vi "Lab Panel V5.22.vi"() -> ()   [LabVIEW 2013] (continued)
                            n2491 = Bundle By Name("Y"=w4658, "t0"=w4656) -> (w4650:waveform(dbl))  [unwired: 1 in]
                            n2492 = Bundle By Name("Y"=w4657, "t0"=w4656) -> (w4649:waveform(dbl))  [unwired: 1 in]
                            n2493 = Build Array(w4655, w4654, w4653, w4652, w4651, w4650, w4649) -> (w4648:waveform(dbl)[])
                            n2494 = TDMS Write(0:w4669, 5:"TEST VALUES", 7:w4640, 9:w4648) -> (4:w4639:refnum<k34>, 6:w4638:string, 15:w4637:errorcluster)  [unwired: 2 in, 1 out]
                            n2495 = TDMS Write(0:w4639, 5:w4638, 7:"TIME", 9:w4635, 11:w4637) -> (15:w4634:errorcluster)  [unwired: 1 in, 3 out]
                            n2496 = local write "data file error"(w4634) -> ()
                          }
                        }
                      }
                    }
                  }
                }
              }
            }
          }
          frame #13 {
            # "display test values on chart"
            n2497 = local read "jig cycle"() -> (w4677:dbl)
            n2498 = local read "on loops"() -> (w4679:dbl)
            n2499 = Add(x=w4679, y=2) -> (x+y=w4676:dbl)
            n2500 = Equal?(x=w4677, y=1) -> (x = y?=w4675:bool)
            n2501 = Equal?(x=w4677, y=w4676) -> (x = y?=w4674:bool)
            n2502 = Or(x=w4675, y=w4674) -> (x .or. y?=w4673:bool)
            "graph flag" <- w4673
            n2503 = global write "Global display 3.vi" "graph flag"(w4673) -> ()
            n2504 = case shown="True" w4673 {
              frame False {
              }
              frame True {
                n2505 = local read "SIG LAB05-1"() -> (w4722:T2)
                n2506 = local read "SIG LAB04-2"() -> (w4723:T2)
                n2507 = local read "SIG LAB05-2"() -> (w4721:T2)
                n2508 = local read "SIG LAB04-1"() -> (w4724:T2)
                n2509 = local read "SIG LAB03-1"() -> (w4726:T2)
                n2510 = local read "SIG LAB03-2"() -> (w4725:T2)
                n2511 = local read "SIG LAB01-1"() -> (w4730:T2)
                n2512 = local read "SIG LAB02-2"() -> (w4727:T2)
                n2513 = local read "SIG LAB02-1"() -> (w4728:T2)
                n2514 = local read "SIG LAB01-2"() -> (w4729:T2)
                n2515 = Unbundle(w4723) -> ("AMPS"=w4713:dbl, "VOLTS"=w4703:dbl, "Tmp Live"=w4693:dbl, "Tmp Neut"=w4683:dbl)  [unwired: 1 out]
                n2516 = Unbundle(w4722) -> ("AMPS"=w4712:dbl, "VOLTS"=w4702:dbl, "Tmp Live"=w4692:dbl, "Tmp Neut"=w4682:dbl)  [unwired: 1 out]
                n2517 = Unbundle(w4721) -> ("AMPS"=w4711:dbl, "VOLTS"=w4701:dbl, "Tmp Live"=w4691:dbl, "Tmp Neut"=w4681:dbl)  [unwired: 1 out]
                n2518 = Unbundle(w4724) -> ("AMPS"=w4714:dbl, "VOLTS"=w4704:dbl, "Tmp Live"=w4694:dbl, "Tmp Neut"=w4684:dbl)  [unwired: 1 out]
                n2519 = Unbundle(w4725) -> ("AMPS"=w4715:dbl, "VOLTS"=w4705:dbl, "Tmp Live"=w4695:dbl, "Tmp Neut"=w4685:dbl)  [unwired: 1 out]
                n2520 = Unbundle(w4726) -> ("AMPS"=w4716:dbl, "VOLTS"=w4706:dbl, "Tmp Live"=w4696:dbl, "Tmp Neut"=w4686:dbl)  [unwired: 1 out]
                n2521 = Unbundle(w4727) -> ("AMPS"=w4717:dbl, "VOLTS"=w4707:dbl, "Tmp Live"=w4697:dbl, "Tmp Neut"=w4687:dbl)  [unwired: 1 out]
                n2522 = Unbundle(w4728) -> ("AMPS"=w4718:dbl, "VOLTS"=w4708:dbl, "Tmp Live"=w4698:dbl, "Tmp Neut"=w4688:dbl)  [unwired: 1 out]
                n2523 = Unbundle(w4730) -> ("AMPS"=w4720:dbl, "VOLTS"=w4710:dbl, "Tmp Live"=w4700:dbl, "Tmp Neut"=w4690:dbl)  [unwired: 1 out]
                n2524 = Unbundle(w4729) -> ("AMPS"=w4719:dbl, "VOLTS"=w4709:dbl, "Tmp Live"=w4699:dbl, "Tmp Neut"=w4689:dbl)  [unwired: 1 out]
                n2525 = stacked-sequence {
                  tunnel: w4720 -> [w4762 _ _]
                  tunnel: w4719 -> [w4761 _ _]
                  tunnel: w4718 -> [w4752 _ _]
                  tunnel: w4717 -> [w4751 _ _]
                  tunnel: w4716 -> [w4741 _ _]
                  tunnel: w4715 -> [w4740 _ _]
                  tunnel: w4714 -> [_ w4785 _]
                  tunnel: w4713 -> [_ w4784 _]
                  tunnel: w4712 -> [_ w4774 _]
                  tunnel: w4711 -> [_ w4773 _]
                  tunnel: w4710 -> [w4759 _ _]
                  tunnel: w4709 -> [w4758 _ _]
                  tunnel: w4708 -> [w4749 _ _]
                  tunnel: w4707 -> [w4748 _ _]
                  tunnel: w4706 -> [w4739 _ _]
                  tunnel: w4705 -> [w4738 _ _]
                  tunnel: w4704 -> [_ w4783 _]
                  tunnel: w4703 -> [_ w4782 _]
                  tunnel: w4702 -> [_ w4772 _]
                  tunnel: w4701 -> [_ w4771 _]
                  tunnel: w4700 -> [w4756 _ _]
                  tunnel: w4699 -> [w4754 _ _]
                  tunnel: w4698 -> [w4745 _ _]
                  tunnel: w4697 -> [w4743 _ _]
                  tunnel: w4696 -> [w4737 _ _]
                  tunnel: w4695 -> [w4735 _ _]
                  tunnel: w4694 -> [_ w4781 _]
                  tunnel: w4693 -> [_ w4779 _]
                  tunnel: w4692 -> [_ w4770 _]
                  tunnel: w4691 -> [_ w4768 _]
                  tunnel: w4690 -> [w4755 _ _]
                  tunnel: w4689 -> [w4753 _ _]
                  tunnel: w4688 -> [w4744 _ _]
                  tunnel: w4687 -> [w4742 _ _]
                  tunnel: w4686 -> [w4736 _ _]
                  tunnel: w4685 -> [w4734 _ _]
                  tunnel: w4684 -> [_ w4780 _]
                  tunnel: w4683 -> [_ w4778 _]
                  tunnel: w4682 -> [_ w4769 _]
                  tunnel: w4681 -> [_ w4767 _]
                  frame #0 {
                    n2526 = Merge Signals(w4762, w4761) -> (→"LAB01 AMPS":dynamicdata)
                    n2527 = Merge Signals(w4759, w4758) -> (→"LAB01 VOLTS":dynamicdata)
                    n2528 = Merge Signals(w4739, w4738) -> (→"LAB03 VOLTS":dynamicdata)
                    n2529 = Merge Signals(w4756, w4755, w4754, w4753) -> (→"LAB01 deg C":dynamicdata)
                    n2530 = Merge Signals(w4752, w4751) -> (→"LAB02 AMPS":dynamicdata)
                    n2531 = Merge Signals(w4745, w4744, w4743, w4742) -> (→"LAB02 deg C":dynamicdata)
                    n2532 = Merge Signals(w4737, w4736, w4735, w4734) -> (→"LAB03 deg C":dynamicdata)
                    n2533 = Merge Signals(w4749, w4748) -> (→"LAB02 VOLTS":dynamicdata)
                    n2534 = Merge Signals(w4741, w4740) -> (→"LAB03 AMPS":dynamicdata)
                  }
                  frame #1 {
                    n2535 = Merge Signals(w4772, w4771) -> (→"LAB05 VOLTS":dynamicdata)
                    n2536 = Merge Signals(w4785, w4784) -> (→"LAB04 AMPS":dynamicdata)
                    n2537 = Merge Signals(w4774, w4773) -> (→"LAB05 AMPS":dynamicdata)
                    n2538 = Merge Signals(w4770, w4769, w4768, w4767) -> (→"LAB05 deg C":dynamicdata)
                    n2539 = Merge Signals(w4781, w4780, w4779, w4778) -> (→"LAB04 deg C":dynamicdata)
                    n2540 = Merge Signals(w4783, w4782) -> (→"LAB04 VOLTS":dynamicdata)
                  }
                  frame #2 {
                    n2541 = local read "LAB05 VOLTS"() -> (w4793:dynamicdata)
                    n2542 = local read "LAB04 VOLTS"() -> (w4794:dynamicdata)
                    n2543 = local read "LAB02 VOLTS"() -> (w4796:dynamicdata)
                    n2544 = local read "LAB03 VOLTS"() -> (w4795:dynamicdata)
                    n2545 = local read "LAB05 AMPS"() -> (w4799:dynamicdata)
                    n2546 = local read "LAB01 VOLTS"() -> (w4797:dynamicdata)
                    n2547 = local read "LAB04 AMPS"() -> (w4800:dynamicdata)
                    n2548 = local read "LAB03 AMPS"() -> (w4801:dynamicdata)
                    n2549 = local read "LAB03 deg C"() -> (w4789:dynamicdata)
                    n2550 = local read "LAB02 AMPS"() -> (w4802:dynamicdata)
                    n2551 = local read "LAB04 deg C"() -> (w4788:dynamicdata)
                    n2552 = local read "LAB05 deg C"() -> (w4787:dynamicdata)
                    n2553 = local read "LAB02 deg C"() -> (w4790:dynamicdata)
                    n2554 = local read "LAB01 deg C"() -> (w4791:dynamicdata)
                    n2555 = local read "LAB01 AMPS"() -> (w4803:dynamicdata)
                    n2556 = Merge Signals(w4791, w4790, w4789, w4788, w4787) -> (w4786:dynamicdata)
                    n2557 = Merge Signals(w4803, w4802, w4801, w4800, w4799) -> (w4798:dynamicdata)
                    n2558 = Merge Signals(w4797, w4796, w4795, w4794, w4793) -> (w4792:dynamicdata)
                    n2559 = global write "Global display 3.vi" "graph volts"(w4792) -> ()
                    n2560 = global write "Global display 3.vi" "graph deg C"(w4786) -> ()
                    n2561 = global write "Global display 3.vi" "graph amps"(w4798) -> ()
                  }
                }
              }
            }
          }
          frame #14 {
            # "check for amps fail"
            # "check for cycle test & temperature rise fail conditions"
            n2562 = local read "on loops"() -> (w4830:dbl)
            n2563 = local read "jig cycle"() -> (w4827:dbl)
            n2564 = local read "jig cycle"() -> (w4832:dbl)
            n2565 = Add(x=w4830, y=3.0) -> (x+y=w4828:dbl)
            n2566 = Equal?(x=w4827, y=w4828) -> (x = y?=w4823:bool)
            n2567 = local read "Fail Loops"() -> (w4804:dbl)
            n2568 = Equal?(x=w4832, y=1.0) -> (x = y?=w4825:bool)
            n2569 = global write "Global 1.vi" "fail count"(w4804) -> ()
            n2570 = stacked-sequence {
              tunnel: w4826 -> [w4835 _ _ _ _ _ _ _ _ _]
              tunnel: w4825 -> [w4836 w4856 w4876 w4896 w4916 w4936 w4956 w4976 w4996 w5016]
              tunnel: w4824 -> [w4833 _ _ _ _ _ _ _ _ _]
              tunnel: w4823 -> [w4834 w4855 w4875 w4895 w4915 w4935 w4955 w4975 w4995 w5015]
              tunnel: w4822 -> [_ w4854 _ _ _ _ _ _ _ _]
              tunnel: w4821 -> [_ w4853 _ _ _ _ _ _ _ _]
              tunnel: w4820 -> [_ _ w4874 _ _ _ _ _ _ _]
              tunnel: w4819 -> [_ _ w4873 _ _ _ _ _ _ _]
              tunnel: w4818 -> [_ _ _ w4894 _ _ _ _ _ _]
              tunnel: w4817 -> [_ _ _ w4893 _ _ _ _ _ _]
              tunnel: w4816 -> [_ _ _ _ w4914 _ _ _ _ _]
              tunnel: w4815 -> [_ _ _ _ w4913 _ _ _ _ _]
              tunnel: w4814 -> [_ _ _ _ _ w4934 _ _ _ _]
              tunnel: w4813 -> [_ _ _ _ _ w4933 _ _ _ _]
              tunnel: w4812 -> [_ _ _ _ _ _ w4954 _ _ _]
              tunnel: w4811 -> [_ _ _ _ _ _ w4953 _ _ _]
              tunnel: w4810 -> [_ _ _ _ _ _ _ w4974 _ _]
              tunnel: w4809 -> [_ _ _ _ _ _ _ w4973 _ _]
              tunnel: w4808 -> [_ _ _ _ _ _ _ _ w4994 _]
              tunnel: w4807 -> [_ _ _ _ _ _ _ _ w4993 _]
              tunnel: w4806 -> [_ _ _ _ _ _ _ _ _ w5014]
              tunnel: w4805 -> [_ _ _ _ _ _ _ _ _ w5013]
              frame #0 {
                # "LAB01-1"
                n2571 = case shown="True" w4833 {
                  tunnel: w4836 -> [_ w4849]
                  tunnel: w4835 -> [_ w4846]
                  tunnel: w4834 -> [_ w4845]
                  frame False {
                  }
                  frame True {
                    n2572 = local read "TEMP START LAB01-1"() -> (w4851:cluster{"TL":dbl, "TN":dbl})
                    n2573 = local read "RESULT LAB01-1"() -> (w4840:bool)
                    n2574 = local read "FAIL LAB01-1"() -> (w4843:cluster{"LO":dbl, "HI":dbl})
                    n2575 = local read "TDMS LAB01-1"() -> (w4850:refnum<k34>)
                    n2576 = local read "SET LAB01-1"() -> (w4847:T5)
                    n2577 = local read "DISP LAB01-1"() -> (w4848:T4)
                    n2578 = local read "SIG LAB01-1"() -> (w4852:T2)
                    n2579 = Bundle("FAIL LAB01-1"=w4843, "SIG LAB01-1"=w4852, "TEMP START LAB01-1"=w4851, "DISP LAB01-1"=w4848, "SET LAB01-1"=w4847, "TDMS LAB01-1"=w4850) -> (w4837:T32)  [unwired: 1 in]
                    n2580 = call "sub vi - cycle&temp fail v7.vi"("Amps Lo?"=w4849, "Input Cluster"=w4837, "SELECT"=w4846, "Amps Hi?"=w4845, "Result In"=w4840) -> ("(FAIL) out"=w4842:cluster{"FAIL LO":dbl, "FAIL HI":dbl}, "(DISP) out"=w4838:T4, "T-RISE"=w4839:cluster{"T-RISE (L)":dbl, "T-RISE (N)":dbl}, "Result Out"=w4841:bool, "file error"=w4844:errorcluster)  [unwired: 10 in]
                    n2581 = local write "TEMP RISE LAB01-1"(w4839) -> ()
                    n2582 = local write "FAIL LAB01-1"(w4842) -> ()
                    n2583 = local write "DISP LAB01-1"(w4838) -> ()
                    n2584 = local write "RESULT LAB01-1"(w4841) -> ()
                    n2585 = local write "data file error"(w4844) -> ()
                  }
                }
              }
              frame #1 {
                # "LAB01-2"
                n2586 = case shown="True" w4854 {
                  tunnel: w4856 -> [_ w4869]
                  tunnel: w4853 -> [_ w4866]
                  tunnel: w4855 -> [_ w4865]
                  frame False {
                  }
                  frame True {
                    n2587 = local read "TEMP START LAB01-2"() -> (w4871:cluster{"TL":dbl, "TN":dbl})
                    n2588 = local read "FAIL LAB01-2"() -> (w4862:cluster{"LO":dbl, "HI":dbl})
                    n2589 = local read "TDMS LAB01-2"() -> (w4870:refnum<k34>)
                    n2590 = local read "SET LAB01-2"() -> (w4867:T5)
                    n2591 = local read "DISP LAB01-2"() -> (w4868:T4)
                    n2592 = local read "RESULT LAB01-2"() -> (w4859:bool)
                    n2593 = local read "SIG LAB01-2"() -> (w4872:T2)
                    n2594 = Bundle("FAIL LAB01-2"=w4862, "SIG LAB01-2"=w4872, "TEMP START LAB01-2"=w4871, "DISP LAB01-2"=w4868, "SET LAB01-2"=w4867, "TDMS LAB01-2"=w4870) -> (w4857:T33)  [unwired: 1 in]
                    n2595 = call "sub vi - cycle&temp fail v7.vi"("Amps Lo?"=w4869, "Input Cluster"=w4857, "SELECT"=w4866, "Amps Hi?"=w4865, "Result In"=w4859) -> ("(FAIL) out"=w4861:cluster{"FAIL LO":dbl, "FAIL HI":dbl}, "(DISP) out"=w4864:T4, "T-RISE"=w4858:cluster{"T-RISE (L)":dbl, "T-RISE (N)":dbl}, "Result Out"=w4860:bool, "file error"=w4863:errorcluster)  [unwired: 10 in]
                    n2596 = local write "TEMP RISE LAB01-2"(w4858) -> ()
                    n2597 = local write "FAIL LAB01-2"(w4861) -> ()
                    n2598 = local write "DISP LAB01-2"(w4864) -> ()
                    n2599 = local write "RESULT LAB01-2"(w4860) -> ()
                    n2600 = local write "data file error"(w4863) -> ()
                  }
                }
              }
              frame #2 {
                # "LAB02-1"
                n2601 = case shown="True" w4874 {
                  tunnel: w4876 -> [_ w4889]
                  tunnel: w4873 -> [_ w4886]
                  tunnel: w4875 -> [_ w4885]
                  frame False {
                  }
                  frame True {
                    n2602 = local read "TEMP START LAB02-1"() -> (w4891:cluster{"TL":dbl, "TN":dbl})
                    n2603 = local read "FAIL LAB02-1"() -> (w4882:cluster{"LO":dbl, "HI":dbl})
                    n2604 = local read "TDMS LAB02-1"() -> (w4890:refnum<k34>)
                    n2605 = local read "SET LAB02-1"() -> (w4887:T5)
                    n2606 = local read "DISP LAB02-1"() -> (w4888:T4)
                    n2607 = local read "SIG LAB02-1"() -> (w4892:T2)
                    n2608 = local read "RESULT LAB02-1"() -> (w4879:bool)
                    n2609 = Bundle("FAIL LAB02-1"=w4882, "SIG LAB02-1"=w4892, "TEMP START LAB02-1"=w4891, "DISP LAB02-1"=w4888, "SET LAB02-1"=w4887, "TDMS LAB02-1"=w4890) -> (w4877:T34)  [unwired: 1 in]
                    n2610 = call "sub vi - cycle&temp fail v7.vi"("Amps Lo?"=w4889, "Input Cluster"=w4877, "SELECT"=w4886, "Amps Hi?"=w4885, "Result In"=w4879) -> ("(FAIL) out"=w4881:cluster{"FAIL LO":dbl, "FAIL HI":dbl}, "(DISP) out"=w4884:T4, "T-RISE"=w4878:cluster{"T-RISE (L)":dbl, "T-RISE (N)":dbl}, "Result Out"=w4880:bool, "file error"=w4883:errorcluster)  [unwired: 10 in]
                    n2611 = local write "TEMP RISE LAB02-1"(w4878) -> ()
                    n2612 = local write "FAIL LAB02-1"(w4881) -> ()
                    n2613 = local write "DISP LAB02-1"(w4884) -> ()
                    n2614 = local write "RESULT LAB02-1"(w4880) -> ()
                    n2615 = local write "data file error"(w4883) -> ()
                  }
                }
              }
              frame #3 {
                # "LAB02-2"
                n2616 = case shown="True" w4894 {
                  tunnel: w4896 -> [_ w4909]
                  tunnel: w4893 -> [_ w4906]
                  tunnel: w4895 -> [_ w4905]
                  frame False {
                  }
                  frame True {
                    n2617 = local read "TEMP START LAB02-2"() -> (w4911:cluster{"TL":dbl, "TN":dbl})
                    n2618 = local read "FAIL LAB02-2"() -> (w4902:cluster{"LO":dbl, "HI":dbl})
                    n2619 = local read "TDMS LAB02-2"() -> (w4910:refnum<k34>)
                    n2620 = local read "SET LAB02-2"() -> (w4907:T5)
                    n2621 = local read "DISP LAB02-2"() -> (w4908:T4)
                    n2622 = local read "SIG LAB02-2"() -> (w4912:T2)
                    n2623 = local read "RESULT LAB02-2"() -> (w4899:bool)
                    n2624 = Bundle("FAIL LAB02-2"=w4902, "SIG LAB02-2"=w4912, "TEMP START LAB02-2"=w4911, "DISP LAB02-2"=w4908, "SET LAB02-2"=w4907, "TDMS LAB02-2"=w4910) -> (w4897:T35)  [unwired: 1 in]
                    n2625 = call "sub vi - cycle&temp fail v7.vi"("Amps Lo?"=w4909, "Input Cluster"=w4897, "SELECT"=w4906, "Amps Hi?"=w4905, "Result In"=w4899) -> ("(FAIL) out"=w4901:cluster{"FAIL LO":dbl, "FAIL HI":dbl}, "(DISP) out"=w4904:T4, "T-RISE"=w4898:cluster{"T-RISE (L)":dbl, "T-RISE (N)":dbl}, "Result Out"=w4900:bool, "file error"=w4903:errorcluster)  [unwired: 10 in]
                    n2626 = local write "TEMP RISE LAB02-2"(w4898) -> ()
                    n2627 = local write "FAIL LAB02-2"(w4901) -> ()
                    n2628 = local write "DISP LAB02-2"(w4904) -> ()
                    n2629 = local write "RESULT LAB02-2"(w4900) -> ()
                    n2630 = local write "data file error"(w4903) -> ()
                  }
                }
              }
              frame #4 {
                # "LAB03-1"
                n2631 = case shown="True" w4914 {
                  tunnel: w4916 -> [_ w4929]
                  tunnel: w4913 -> [_ w4926]
                  tunnel: w4915 -> [_ w4925]
                  frame False {
                  }
                  frame True {
                    n2632 = local read "TEMP START LAB03-1"() -> (w4931:cluster{"TL":dbl, "TN":dbl})
                    n2633 = local read "FAIL LAB03-1"() -> (w4922:cluster{"LO":dbl, "HI":dbl})
                    n2634 = local read "TDMS LAB03-1"() -> (w4930:refnum<k34>)
                    n2635 = local read "SET LAB03-1"() -> (w4927:T5)
                    n2636 = local read "DISP LAB03-1"() -> (w4928:T4)
                    n2637 = local read "SIG LAB03-1"() -> (w4932:T2)
                    n2638 = local read "RESULT LAB03-1"() -> (w4919:bool)
                    n2639 = Bundle("FAIL LAB03-1"=w4922, "SIG LAB03-1"=w4932, "TEMP START LAB03-1"=w4931, "DISP LAB03-1"=w4928, "SET LAB03-1"=w4927, "TDMS LAB03-1"=w4930) -> (w4917:T36)  [unwired: 1 in]
                    n2640 = call "sub vi - cycle&temp fail v7.vi"("Amps Lo?"=w4929, "Input Cluster"=w4917, "SELECT"=w4926, "Amps Hi?"=w4925, "Result In"=w4919) -> ("(FAIL) out"=w4921:cluster{"FAIL LO":dbl, "FAIL HI":dbl}, "(DISP) out"=w4924:T4, "T-RISE"=w4918:cluster{"T-RISE (L)":dbl, "T-RISE (N)":dbl}, "Result Out"=w4920:bool, "file error"=w4923:errorcluster)  [unwired: 10 in]
                    n2641 = local write "TEMP RISE LAB03-1"(w4918) -> ()
                    n2642 = local write "FAIL LAB03-1"(w4921) -> ()
                    n2643 = local write "DISP LAB03-1"(w4924) -> ()
                    n2644 = local write "RESULT LAB03-1"(w4920) -> ()
                    n2645 = local write "data file error"(w4923) -> ()
                  }
                }
              }
              frame #5 {
                # "LAB03-2"
                n2646 = case shown="True" w4934 {
                  tunnel: w4936 -> [_ w4949]
                  tunnel: w4933 -> [_ w4946]
                  tunnel: w4935 -> [_ w4945]
                  frame False {
                  }
                  frame True {
                    n2647 = local read "TEMP START LAB03-2"() -> (w4951:cluster{"TL":dbl, "TN":dbl})
                    n2648 = local read "FAIL LAB03-2"() -> (w4942:cluster{"LO":dbl, "HI":dbl})
                    n2649 = local read "TDMS LAB03-2"() -> (w4950:refnum<k34>)
                    n2650 = local read "SET LAB03-2"() -> (w4947:T5)
                    n2651 = local read "DISP LAB03-2"() -> (w4948:T4)
                    n2652 = local read "RESULT LAB03-2"() -> (w4939:bool)
                    n2653 = local read "SIG LAB03-2"() -> (w4952:T2)
                    n2654 = Bundle("FAIL LAB03-2"=w4942, "SIG LAB03-2"=w4952, "TEMP START LAB03-2"=w4951, "DISP LAB03-2"=w4948, "SET LAB03-2"=w4947, "TDMS LAB03-2"=w4950) -> (w4937:T37)  [unwired: 1 in]
                    n2655 = call "sub vi - cycle&temp fail v7.vi"("Amps Lo?"=w4949, "Input Cluster"=w4937, "SELECT"=w4946, "Amps Hi?"=w4945, "Result In"=w4939) -> ("(FAIL) out"=w4941:cluster{"FAIL LO":dbl, "FAIL HI":dbl}, "(DISP) out"=w4944:T4, "T-RISE"=w4938:cluster{"T-RISE (L)":dbl, "T-RISE (N)":dbl}, "Result Out"=w4940:bool, "file error"=w4943:errorcluster)  [unwired: 10 in]
                    n2656 = local write "FAIL LAB03-2"(w4941) -> ()
                    n2657 = local write "TEMP RISE LAB03-2"(w4938) -> ()
                    n2658 = local write "DISP LAB03-2"(w4944) -> ()
                    n2659 = local write "RESULT LAB03-2"(w4940) -> ()
                    n2660 = local write "data file error"(w4943) -> ()
                  }
                }
              }
              frame #6 {
                # "LAB04-1"
                n2661 = case shown="True" w4954 {
                  tunnel: w4956 -> [_ w4969]
                  tunnel: w4953 -> [_ w4966]
                  tunnel: w4955 -> [_ w4965]
                  frame False {
                  }
                  frame True {
                    n2662 = local read "TEMP START LAB04-1"() -> (w4971:cluster{"TL":dbl, "TN":dbl})
                    n2663 = local read "FAIL LAB04-1"() -> (w4962:cluster{"LO":dbl, "HI":dbl})
                    n2664 = local read "TDMS LAB04-1"() -> (w4970:refnum<k34>)
                    n2665 = local read "SET LAB04-1"() -> (w4967:T5)
                    n2666 = local read "DISP LAB04-1"() -> (w4968:T4)
                    n2667 = local read "SIG LAB04-1"() -> (w4972:T2)
                    n2668 = local read "RESULT LAB04-1"() -> (w4959:bool)
                    n2669 = Bundle("FAIL LAB04-1"=w4962, "SIG LAB04-1"=w4972, "TEMP START LAB04-1"=w4971, "DISP LAB04-1"=w4968, "SET LAB04-1"=w4967, "TDMS LAB04-1"=w4970) -> (w4957:T38)  [unwired: 1 in]
                    n2670 = call "sub vi - cycle&temp fail v7.vi"("Amps Lo?"=w4969, "Input Cluster"=w4957, "SELECT"=w4966, "Amps Hi?"=w4965, "Result In"=w4959) -> ("(FAIL) out"=w4961:cluster{"FAIL LO":dbl, "FAIL HI":dbl}, "(DISP) out"=w4964:T4, "T-RISE"=w4958:cluster{"T-RISE (L)":dbl, "T-RISE (N)":dbl}, "Result Out"=w4960:bool, "file error"=w4963:errorcluster)  [unwired: 10 in]
                    n2671 = local write "TEMP RISE LAB04-1"(w4958) -> ()
                    n2672 = local write "FAIL LAB04-1"(w4961) -> ()
                    n2673 = local write "DISP LAB04-1"(w4964) -> ()
                    n2674 = local write "RESULT LAB04-1"(w4960) -> ()
                    n2675 = local write "data file error"(w4963) -> ()
                  }
                }
              }
              frame #7 {
                # "LAB04-2"
                n2676 = case shown="True" w4974 {
                  tunnel: w4976 -> [_ w4989]
                  tunnel: w4973 -> [_ w4986]
                  tunnel: w4975 -> [_ w4985]
                  frame False {
                  }
                  frame True {
                    n2677 = local read "TEMP START LAB04-2"() -> (w4991:cluster{"TL":dbl, "TN":dbl})
                    n2678 = local read "FAIL LAB04-2"() -> (w4982:cluster{"LO":dbl, "HI":dbl})
                    n2679 = local read "TDMS LAB04-2"() -> (w4990:refnum<k34>)
                    n2680 = local read "SET LAB04-2"() -> (w4987:T5)
                    n2681 = local read "DISP LAB04-2"() -> (w4988:T4)
                    n2682 = local read "SIG LAB04-2"() -> (w4992:T2)
                    n2683 = local read "RESULT LAB04-2"() -> (w4979:bool)
                    n2684 = Bundle("FAIL LAB04-2"=w4982, "SIG LAB04-2"=w4992, "TEMP START LAB04-2"=w4991, "DISP LAB04-2"=w4988, "SET LAB04-2"=w4987, "TDMS LAB04-2"=w4990) -> (w4977:T39)  [unwired: 1 in]
                    n2685 = call "sub vi - cycle&temp fail v7.vi"("Amps Lo?"=w4989, "Input Cluster"=w4977, "SELECT"=w4986, "Amps Hi?"=w4985, "Result In"=w4979) -> ("(FAIL) out"=w4981:cluster{"FAIL LO":dbl, "FAIL HI":dbl}, "(DISP) out"=w4984:T4, "T-RISE"=w4978:cluster{"T-RISE (L)":dbl, "T-RISE (N)":dbl}, "Result Out"=w4980:bool, "file error"=w4983:errorcluster)  [unwired: 10 in]
                    n2686 = local write "TEMP RISE LAB04-2"(w4978) -> ()
                    n2687 = local write "FAIL LAB04-2"(w4981) -> ()
                    n2688 = local write "DISP LAB04-2"(w4984) -> ()
                    n2689 = local write "RESULT LAB04-2"(w4980) -> ()
                    n2690 = local write "data file error"(w4983) -> ()
                  }
                }
              }
              frame #8 {
                # "LAB05-1"
                n2691 = case shown="True" w4994 {
                  tunnel: w4996 -> [_ w5009]
                  tunnel: w4993 -> [_ w5006]
                  tunnel: w4995 -> [_ w5005]
                  frame False {
                  }
                  frame True {
                    n2692 = local read "TEMP START LAB05-1"() -> (w5011:cluster{"TL":dbl, "TN":dbl})
                    n2693 = local read "FAIL LAB05-1"() -> (w5002:cluster{"LO":dbl, "HI":dbl})
                    n2694 = local read "TDMS LAB05-1"() -> (w5010:refnum<k34>)
                    n2695 = local read "SET LAB05-1"() -> (w5007:T5)
                    n2696 = local read "DISP LAB05-1"() -> (w5008:T4)
                    n2697 = local read "SIG LAB05-1"() -> (w5012:T2)
                    n2698 = local read "RESULT LAB05-1"() -> (w4999:bool)
                    n2699 = Bundle("FAIL LAB05-1"=w5002, "SIG LAB05-1"=w5012, "TEMP START LAB05-1"=w5011, "DISP LAB05-1"=w5008, "SET LAB05-1"=w5007, "TDMS LAB05-1"=w5010) -> (w4997:T40)  [unwired: 1 in]
                    n2700 = call "sub vi - cycle&temp fail v7.vi"("Amps Lo?"=w5009, "Input Cluster"=w4997, "SELECT"=w5006, "Amps Hi?"=w5005, "Result In"=w4999) -> ("(FAIL) out"=w5001:cluster{"FAIL LO":dbl, "FAIL HI":dbl}, "(DISP) out"=w5004:T4, "T-RISE"=w4998:cluster{"T-RISE (L)":dbl, "T-RISE (N)":dbl}, "Result Out"=w5000:bool, "file error"=w5003:errorcluster)  [unwired: 10 in]
                    n2701 = local write "TEMP RISE LAB05-1"(w4998) -> ()
                    n2702 = local write "FAIL LAB05-1"(w5001) -> ()
                    n2703 = local write "DISP LAB05-1"(w5004) -> ()
                    n2704 = local write "RESULT LAB05-1"(w5000) -> ()
                    n2705 = local write "data file error"(w5003) -> ()
                  }
                }
              }
              frame #9 {
                # "LAB05-2"
                n2706 = case shown="True" w5014 {
                  tunnel: w5016 -> [_ w5029]
                  tunnel: w5013 -> [_ w5026]
                  tunnel: w5015 -> [_ w5025]
                  frame False {
                  }
                  frame True {
                    n2707 = local read "TEMP START LAB05-2"() -> (w5031:cluster{"TL":dbl, "TN":dbl})
                    n2708 = local read "FAIL LAB05-2"() -> (w5022:cluster{"LO":dbl, "HI":dbl})
                    n2709 = local read "TDMS LAB05-2"() -> (w5030:refnum<k34>)
                    n2710 = local read "SET LAB05-2"() -> (w5027:T5)
                    n2711 = local read "DISP LAB05-2"() -> (w5028:T4)
                    n2712 = local read "SIG LAB05-2"() -> (w5032:T2)
                    n2713 = local read "RESULT LAB05-2"() -> (w5019:bool)
                    n2714 = Bundle("FAIL LAB05-2"=w5022, "SIG LAB05-2"=w5032, "TEMP START LAB05-2"=w5031, "DISP LAB05-2"=w5028, "SET LAB05-2"=w5027, "TDMS LAB05-2"=w5030) -> (w5017:T41)  [unwired: 1 in]
                    n2715 = call "sub vi - cycle&temp fail v7.vi"("Amps Lo?"=w5029, "Input Cluster"=w5017, "SELECT"=w5026, "Amps Hi?"=w5025, "Result In"=w5019) -> ("(FAIL) out"=w5021:cluster{"FAIL LO":dbl, "FAIL HI":dbl}, "(DISP) out"=w5024:T4, "T-RISE"=w5018:cluster{"T-RISE (L)":dbl, "T-RISE (N)":dbl}, "Result Out"=w5020:bool, "file error"=w5023:errorcluster)  [unwired: 10 in]
                    n2716 = local write "TEMP RISE LAB05-2"(w5018) -> ()
                    n2717 = local write "FAIL LAB05-2"(w5021) -> ()
                    n2718 = local write "DISP LAB05-2"(w5024) -> ()
                    n2719 = local write "RESULT LAB05-2"(w5020) -> ()
                    n2720 = local write "data file error"(w5023) -> ()
                  }
                }
              }
            }
          }
          frame #15 {
            # "run calibration routine"
            n2721 = local read "SET (cal)"() -> (w5033:bool)
            n2722 = case shown="True" w5033 {
              frame False {
              }
              frame True {
                n2723 = stacked-sequence {
                  seq-local: [w5034 _ _] -> [_ w5036 _]
                  frame #0 {
                    n2724 = call "CALIBRATION PASSWORD"() -> ("PASSWORD"=w5034:string)  [unwired: 17 in, 2 out]
                  }
                  frame #1 {
                    n2725 = Equal?(x=w5036, y="7777") -> (x = y?=w5035:bool)
                    n2726 = case shown="True" w5035 {
                      frame False {
                      }
                      frame True {
                        n2727 = stacked-sequence {
                          frame #0 {
                            n2728 = local read "Temp Test Cal"() -> (w5038:dbl)
                            n2729 = call "sub vi - calibration v1.vi"("Temp Test Cal"=w5038) -> ()  [unwired: 11 in]
                          }
                          frame #1 {
                            n2730 = call "sub vi - get calibration values v1.vi"() -> ("TEMP REF CAL"=w5039:dbl, "LAB01 (CAL)"=w5044:T14, "LAB02 (CAL)"=w5043:T15, "LAB03 (CAL)"=w5042:T14, "LAB04 (CAL)"=w5041:T14, "calibration file error out"=w5045:errorcluster, "LAB05 (CAL)"=w5040:T14)  [unwired: 9 in]
                            n2731 = local write "TEMP REF cal"(w5039) -> ()
                            n2732 = local write "cal file error out"(w5045) -> ()
                            n2733 = local write "CAL LAB04"(w5041) -> ()
                            n2734 = local write "CAL LAB05"(w5040) -> ()
                            n2735 = local write "CAL LAB01"(w5044) -> ()
                            n2736 = local write "CAL LAB02"(w5043) -> ()
                            n2737 = local write "CAL LAB03"(w5042) -> ()
                          }
                        }
                      }
                    }
                  }
                  frame #2 {
                    n2738 = local write "SET (cal)"(FALSE) -> ()
                  }
                }
              }
            }
          }
          frame #16 {
            # "save certain settings to file"
            n2739 = String To Path(string="c:\\crabtree\\Set Up\\") -> (path=w5048:path)
            n2740 = Build Path(base path=w5048, name or relative path="settings.bin") -> (appended path=w5050:path)
            n2741 = Build Path(base path=w5048, name or relative path="mail.bin") -> (appended path=w5047:path)
            n2742 = Create Folder(path (use dialog)=w5048) -> (error out=w5053:errorcluster)  [unwired: 2 in, 2 out]
            n2743 = call <vilib>:"Clear Errors.vi"("error in (no error)"=w5053) -> ()  [unwired: 6 in, 1 out]
            n2744 = stacked-sequence {
              seq-local: [w5066 _] -> [_ w5079]
              tunnel: w5050 -> [_ w5080]
              tunnel: w5047 -> [_ w5078]
              frame #0 {
                n2745 = local read "C drive data root dir"() -> (w5065:path)
                n2746 = local read "Select COM port"() -> (w5062:refnum<visa-resource-name>)
                n2747 = local read "Network Directory"() -> (w5071:path)
                n2748 = local read "SET LAB05-2"() -> (w5070:T5)
                n2749 = local read "SET LAB05-1"() -> (w5069:T5)
                n2750 = local read "SET LAB04-2"() -> (w5068:T5)
                n2751 = local read "SET LAB03-2"() -> (w5072:T5)
                n2752 = local read "SET LAB04-1"() -> (w5067:T5)
                n2753 = local read "SET LAB03-1"() -> (w5073:T5)
                n2754 = local read "SET LAB02-2"() -> (w5074:T5)
                n2755 = local read "SET LAB02-1"() -> (w5075:T5)
                n2756 = local read "Temp Delay Lps"() -> (w5061:dbl)
                n2757 = local read "Amps Fail level"() -> (w5057:dbl)
                n2758 = local read "SET LAB01-2"() -> (w5076:T5)
                n2759 = local read "Temp Test Cal"() -> (w5058:dbl)
                n2760 = local read "SET LAB01-1"() -> (w5077:T5)
                n2761 = local read "Mail Test File To:"() -> (w5056:string)
                n2762 = local read "Temp Value"() -> (w5060:dbl)
                n2763 = local read "Fail Loops"() -> (w5059:dbl)
                n2764 = local read "Total USB resets"() -> (w5054:dbl)
                n2765 = local read "Mail Test Fail"() -> (w5055:bool)
                n2766 = local read "RATE (Hz)"() -> (w5064:dbl)
                n2767 = local read "SAMPLES"() -> (w5063:dbl)
                n2768 = Bundle("SET LAB01-1"=w5077, "SET LAB01-2"=w5076, "SET LAB02-1"=w5075, "SET LAB02-2"=w5074, "SET LAB03-1"=w5073, "SET LAB03-2"=w5072, "SET LAB04-1"=w5067, "SET LAB04-2"=w5068, "SET LAB05-1"=w5069, "SET LAB05-2"=w5070, "Network Directory"=w5071, "C drive data root dir"=w5065, "RATE (Hz)"=w5064, "SAMPLES"=w5063, "Select COM port"=w5062, "Temp Delay Lps"=w5061, "Temp Value"=w5060, "Fail Loops"=w5059, "Temp Test Cal"=w5058, "Amps Fail level"=w5057, "Mail Test File To:"=w5056, "Mail Test Fail"=w5055, "Total USB resets"=w5054) -> (w5066:T22)  [unwired: 1 in]
              }
              frame #1 {
                n2769 = event shown="[1] \"SET LAB01-1\", \"SET LAB01-2\", \"SET LAB02-1\", \"SET LAB02-2\", \"SET LAB03-1\", \"SET LAB03-2\", \"SET LAB04-1\", \"SET LAB04-2\", \"SET LAB05-1\", \"SET LAB05-2\", \"Network Directory\", \"C drive data root dir\", \"RATE (Hz)\", \"SAMPLES\", \"Select COM port\", \"Temp Delay Lps\", \"Temp Value\", \"Fail Loops\", \"Temp Test Cal\", \"Amps Fail level\", \"Mail Test File To:\", \"Mail Test Fail\": Value Change" {
                  selector: _ -> [_ _ _]
                  dyn-events: _ -> [_ _ _]
                  timeout: 10.0 -> [_ _ _]
                  tunnel: w5080 -> [_ w5082 _]
                  tunnel: w5079 -> [_ w5083 _]
                  tunnel: w5078 -> [_ _ w5094]
                  event Timeout {
                    n2770 = event-data() -> ()  [unwired: 1 in, 3 out]
                  }
                  event "SET LAB01-1", "SET LAB01-2", "SET LAB02-1", "SET LAB02-2", "SET LAB03-1", "SET LAB03-2", "SET LAB04-1", "SET LAB04-2", "SET LAB05-1", "SET LAB05-2", "Network Directory", "C drive data root dir", "RATE (Hz)", "SAMPLES", "Select COM port", "Temp Delay Lps", "Temp Value", "Fail Loops", "Temp Test Cal", "Amps Fail level", "Mail Test File To:", "Mail Test Fail": Value Change {
                    n2771 = event-data() -> ()  [unwired: 1 in, 6 out]
                    n2772 = Open/Create/Replace File(file path (use dialog)=w5082, operation (0:open)=T21."replace or create") -> (refnum out=w5088:refnum<file>, error out=w5087:errorcluster)  [unwired: 4 in, 1 out]
                    n2773 = Write to Binary File(file (use dialog)=w5088, data=w5083, error in=w5087) -> (refnum out=w5086:refnum<file>, error out=w5085:errorcluster)  [unwired: 3 in, 1 out]
                    n2774 = Close File(refnum=w5086, error in=w5085) -> (error out=w5084:errorcluster)  [unwired: 1 out]
                    n2775 = local write "data file error"(w5084) -> ()
                  }
                  event "MAIL SETTINGS.OUT SERVER ADDRESS", "MAIL SETTINGS.FROM ACCOUNT", "MAIL SETTINGS.USER NAME", "MAIL SETTINGS.PASSWORD", "Auto Mail Send", "TO (string):": Value Change {
                    n2776 = event-data() -> ()  [unwired: 1 in, 6 out]
                    n2777 = local read "MAIL SETTINGS"() -> (w5093:T7)
                    n2778 = local read "Auto Mail Send"() -> (w5091:bool)
                    n2779 = local read "TO (string):"() -> (w5090:string)
                    n2780 = Open/Create/Replace File(file path (use dialog)=w5094, operation (0:open)=T21."replace or create") -> (refnum out=w5099:refnum<file>, error out=w5098:errorcluster)  [unwired: 4 in, 1 out]
                    n2781 = Bundle("MAIL SETTINGS"=w5093, "Auto Mail Send"=w5091, "TO (string):"=w5090) -> (w5092:T42)  [unwired: 1 in]
                    n2782 = Write to Binary File(file (use dialog)=w5099, data=w5092, error in=w5098) -> (refnum out=w5097:refnum<file>, error out=w5096:errorcluster)  [unwired: 3 in, 1 out]
                    n2783 = Close File(refnum=w5097, error in=w5096) -> (error out=w5095:errorcluster)  [unwired: 1 out]
                    n2784 = local write "data file error"(w5095) -> ()
                  }
                }
              }
            }
          }
          frame #17 {
            # "mail control"
            n2785 = local read "MAIL SETTINGS"() -> (w5116:T7)
            n2786 = local read "Auto Mail Send"() -> (w5102:bool)
            n2787 = Unbundle(w5116) -> ("OUT SERVER ADDRESS"=w5115:string, "FROM ACCOUNT"=w5114:string, "TEST MAIL"=w5113:bool)  [unwired: 4 out]
            n2788 = stacked-sequence {
              tunnel: "TO (string):" -> [_ w5155]
              tunnel: w5116 -> [w5121 w5154]
              tunnel: w5115 -> [w5120 w5153]
              tunnel: w5114 -> [w5119 w5152]
              tunnel: w5113 -> [w5118 _]
              tunnel: w5102 -> [_ w5151]
              tunnel: w5112 -> [_ w5150]
              tunnel: w5111 -> [_ w5149]
              tunnel: w5110 -> [_ w5148]
              tunnel: w5109 -> [_ w5147]
              tunnel: w5108 -> [_ w5146]
              tunnel: w5107 -> [_ w5145]
              tunnel: w5106 -> [_ w5144]
              tunnel: w5105 -> [_ w5143]
              tunnel: w5104 -> [_ w5142]
              tunnel: w5103 -> [_ w5141]
              tunnel: "TO (string):" -> [w5117 _]
              frame #0 {
                # "mail test"
                n2789 = case shown="True" w5118 {
                  tunnel: w5121 -> [_ w5125]
                  tunnel: w5117 -> [_ w5124]
                  tunnel: w5120 -> [_ w5123]
                  tunnel: w5119 -> [_ w5122]
                  frame False {
                  }
                  frame True {
                    n2790 = stacked-sequence {
                      seq-local: [_ _ w5135 _] -> [_ _ _ w5136]
                      tunnel: w5125 -> [w5128 _ _ w5140]
                      tunnel: w5124 -> [_ _ w5133 _]
                      tunnel: w5123 -> [_ _ w5131 _]
                      tunnel: w5122 -> [_ _ w5132 _]
                      frame #0 {
                        n2791 = Bundle(cluster=w5128, "TEST MAIL STATUS"="TEST START") -> (w5126:T7)  [unwired: 6 in]
                        n2792 = local write "MAIL SETTINGS"(w5126) -> ()
                      }
                      frame #1 {
                        n2793 = Wait (ms)(milliseconds to wait=500) -> ()  [unwired: 1 out]
                      }
                      frame #2 {
                        n2794 = call "sub vi - send mail v5.vi"("TO:"=w5133, "subject"="MAIL TEST FROM LAB PANEL", "from"=w5132, "out going server"=w5131, "message"="TEST MESSAGE") -> ("error out"=w5135:errorcluster)  [unwired: 10 in]
                      }
                      frame #3 {
                        n2795 = Bundle(cluster=w5140, "TEST MAIL"=FALSE, "TEST MAIL STATUS"="TEST END", "mail error"=w5136) -> (w5138:T7)  [unwired: 4 in]
                        n2796 = local write "MAIL SETTINGS"(w5138) -> ()
                      }
                    }
                  }
                }
              }
              frame #1 {
                # "mail report"
                n2797 = stacked-sequence {
                  seq-local: [_ w5198 _ _] -> [_ _ _ w5388]
                  seq-local: [_ _ w5301 _] -> [_ _ _ w5378]
                  seq-local: [w5165 _ _ _] -> [_ w5215 _ _]
                  seq-local: [w5164 _ _ _] -> [_ w5214 _ _]
                  seq-local: [w5162 _ _ _] -> [_ w5212 _ _]
                  seq-local: [w5163 _ _ _] -> [_ w5213 _ _]
                  seq-local: [w5161 _ _ _] -> [_ w5211 _ _]
                  seq-local: [w5160 _ _ _] -> [_ w5206 _ _]
                  seq-local: [w5159 _ _ _] -> [_ w5207 _ _]
                  seq-local: [w5158 _ _ _] -> [_ w5208 _ _]
                  seq-local: [w5157 _ _ _] -> [_ w5209 _ _]
                  seq-local: [w5156 _ _ _] -> [_ w5210 _ _]
                  tunnel: w5155 -> [_ _ _ w5389]
                  tunnel: w5154 -> [_ _ _ w5372]
                  tunnel: w5153 -> [_ _ _ w5386]
                  tunnel: w5152 -> [_ _ _ w5385]
                  tunnel: w5151 -> [w5196 _ _ w5380]
                  tunnel: w5150 -> [_ _ w5331 _]
                  tunnel: w5149 -> [_ _ w5328 _]
                  tunnel: w5148 -> [_ _ w5327 _]
                  tunnel: w5147 -> [_ _ w5326 _]
                  tunnel: w5146 -> [_ _ w5325 _]
                  tunnel: w5145 -> [_ _ w5324 _]
                  tunnel: w5144 -> [_ _ w5323 _]
                  tunnel: w5143 -> [_ _ w5322 _]
                  tunnel: w5142 -> [_ _ w5321 _]
                  tunnel: w5141 -> [_ _ w5320 _]
                  frame #0 {
                    n2798 = case shown="False" w5196 {
                      frame False {
                        n2799 = local write "mail control"("") -> ()
                      }
                      frame True {
                      }
                    }
                    n2800 = local read "SET LAB01-1"() -> (w5195:T5)
                    n2801 = local read "SET LAB01-2"() -> (w5194:T5)
                    n2802 = local read "SET LAB02-1"() -> (w5193:T5)
                    n2803 = local read "SET LAB02-2"() -> (w5192:T5)
                    n2804 = local read "SET LAB03-1"() -> (w5191:T5)
                    n2805 = local read "SET LAB04-1"() -> (w5189:T5)
                    n2806 = local read "SET LAB05-1"() -> (w5187:T5)
                    n2807 = local read "SET LAB03-2"() -> (w5190:T5)
                    n2808 = local read "SET LAB04-2"() -> (w5188:T5)
                    n2809 = local read "SET LAB05-2"() -> (w5186:T5)
                    n2810 = Unbundle(w5191) -> ("DESCRIPTION"=w5171:string)  [unwired: 4 out]
                    n2811 = Unbundle(w5190) -> ("DESCRIPTION"=w5170:string)  [unwired: 4 out]
                    n2812 = Unbundle(w5189) -> ("DESCRIPTION"=w5169:string)  [unwired: 4 out]
                    n2813 = Unbundle(w5186) -> ("DESCRIPTION"=w5166:string)  [unwired: 4 out]
                    n2814 = Unbundle(w5192) -> ("DESCRIPTION"=w5172:string)  [unwired: 4 out]
                    n2815 = Unbundle(w5188) -> ("DESCRIPTION"=w5168:string)  [unwired: 4 out]
                    n2816 = Unbundle(w5195) -> ("DESCRIPTION"=w5184:string)  [unwired: 4 out]
                    n2817 = Unbundle(w5193) -> ("DESCRIPTION"=w5173:string)  [unwired: 4 out]
                    n2818 = Unbundle(w5187) -> ("DESCRIPTION"=w5167:string)  [unwired: 4 out]
                    n2819 = Unbundle(w5194) -> ("DESCRIPTION"=w5174:string)  [unwired: 4 out]
                    n2820 = Concatenate Strings("[LAB05-2/", w5166) -> (w5156:string)
                    n2821 = Concatenate Strings("[LAB05-1/", w5167) -> (w5157:string)
                    n2822 = Concatenate Strings("[LAB04-2/", w5168) -> (w5158:string)
                    n2823 = Concatenate Strings("[LAB03-2/", w5170) -> (w5160:string)
                    n2824 = Concatenate Strings("[LAB04-1/", w5169) -> (w5159:string)
                    n2825 = Concatenate Strings("[LAB03-1/", w5171) -> (w5161:string)
                    n2826 = Concatenate Strings("[LAB01-2/", w5174) -> (w5164:string)
                    n2827 = Concatenate Strings("[LAB02-2/", w5172) -> (w5162:string)
                    n2828 = Concatenate Strings("[LAB01-1/", w5184) -> (w5165:string)
                    n2829 = Concatenate Strings("[LAB02-1/", w5173) -> (w5163:string)
                  }
                  frame #1 {
                    w5219 = "/"
                    w5220 = 2.0
                    n2830 = local read "DISP LAB01-2"() -> (w5299:T4)
                    n2831 = local read "DISP LAB01-1"() -> (w5300:T4)
                    n2832 = local read "DISP LAB02-1"() -> (w5298:T4)
                    n2833 = local read "DISP LAB03-2"() -> (w5295:T4)
                    n2834 = local read "DISP LAB02-2"() -> (w5297:T4)
                    n2835 = local read "DISP LAB03-1"() -> (w5296:T4)
                    n2836 = local read "DISP LAB04-2"() -> (w5293:T4)
                    n2837 = local read "DISP LAB04-1"() -> (w5294:T4)
                    n2838 = local read "DISP LAB05-1"() -> (w5292:T4)
                    n2839 = local read "DISP LAB05-2"() -> (w5291:T4)
                    n2840 = Unbundle(w5299) -> ("CYCLE"=w5283:dbl, "MINS"=w5282:dbl, "STATUS"=w5279:string)
                    n2841 = Unbundle(w5300) -> ("CYCLE"=w5288:dbl, "MINS"=w5287:dbl, "STATUS"=w5284:string)
                    n2842 = Unbundle(w5298) -> ("CYCLE"=w5276:dbl, "MINS"=w5275:dbl, "STATUS"=w5274:string)
                    n2843 = Unbundle(w5295) -> ("CYCLE"=w5263:dbl, "MINS"=w5262:dbl, "STATUS"=w5259:string)
                    n2844 = Unbundle(w5296) -> ("CYCLE"=w5268:dbl, "MINS"=w5267:dbl, "STATUS"=w5264:string)
                    n2845 = Unbundle(w5297) -> ("CYCLE"=w5273:dbl, "MINS"=w5272:dbl, "STATUS"=w5269:string)
                    n2846 = Unbundle(w5294) -> ("CYCLE"=w5258:dbl, "MINS"=w5257:dbl, "STATUS"=w5254:string)
                    n2847 = Unbundle(w5293) -> ("CYCLE"=w5253:dbl, "MINS"=w5252:dbl, "STATUS"=w5249:string)
                    n2848 = Unbundle(w5292) -> ("CYCLE"=w5248:dbl, "MINS"=w5247:dbl, "STATUS"=w5244:string)
                    n2849 = Unbundle(w5291) -> ("CYCLE"=w5290:dbl, "MINS"=w5289:dbl, "STATUS"=w5241:string)
                    n2850 = Number To Decimal String(number=w5276) -> (decimal integer string=w5278:string)  [unwired: 1 in]
                    n2851 = Number To Decimal String(number=w5273) -> (decimal integer string=w5271:string)  [unwired: 1 in]
                    n2852 = Number To Decimal String(number=w5268) -> (decimal integer string=w5266:string)  [unwired: 1 in]
                    n2853 = Number To Decimal String(number=w5283) -> (decimal integer string=w5281:string)  [unwired: 1 in]
                    n2854 = Number To Decimal String(number=w5263) -> (decimal integer string=w5261:string)  [unwired: 1 in]
                    n2855 = Number To Decimal String(number=w5288) -> (decimal integer string=w5286:string)  [unwired: 1 in]
                    n2856 = Number To Decimal String(number=w5290) -> (decimal integer string=w5243:string)  [unwired: 1 in]
                    n2857 = Number To Decimal String(number=w5258) -> (decimal integer string=w5256:string)  [unwired: 1 in]
                    n2858 = Number To Decimal String(number=w5253) -> (decimal integer string=w5251:string)  [unwired: 1 in]
                    n2859 = Number To Decimal String(number=w5248) -> (decimal integer string=w5246:string)  [unwired: 1 in]
                    n2860 = Number To Fractional String(number=w5275, precision (6)=w5220) -> (F-format string=w5277:string)  [unwired: 2 in]
                    n2861 = Number To Fractional String(number=w5262, precision (6)=w5220) -> (F-format string=w5260:string)  [unwired: 2 in]
                    n2862 = Number To Fractional String(number=w5272, precision (6)=w5220) -> (F-format string=w5270:string)  [unwired: 2 in]
                    n2863 = Number To Fractional String(number=w5267, precision (6)=w5220) -> (F-format string=w5265:string)  [unwired: 2 in]
                    n2864 = Number To Fractional String(number=w5252, precision (6)=w5220) -> (F-format string=w5250:string)  [unwired: 2 in]
                    n2865 = Number To Fractional String(number=w5257, precision (6)=w5220) -> (F-format string=w5255:string)  [unwired: 2 in]
                    n2866 = Number To Fractional String(number=w5282, precision (6)=w5220) -> (F-format string=w5280:string)  [unwired: 2 in]
                    n2867 = Number To Fractional String(number=w5247, precision (6)=w5220) -> (F-format string=w5245:string)  [unwired: 2 in]
                    n2868 = Number To Fractional String(number=w5287, precision (6)=w5220) -> (F-format string=w5285:string)  [unwired: 2 in]
                    n2869 = Number To Fractional String(number=w5289, precision (6)=w5220) -> (F-format string=w5242:string)  [unwired: 2 in]
                    n2870 = Concatenate Strings(w5219, w5261, w5219, w5260, w5219, w5259) -> (w5235:string)
                    n2871 = Concatenate Strings(w5219, w5256, w5219, w5255, w5219, w5254) -> (w5234:string)
                    n2872 = Concatenate Strings(w5219, w5251, w5219, w5250, w5219, w5249) -> (w5233:string)
                    n2873 = Concatenate Strings(w5219, w5246, w5219, w5245, w5219, w5244) -> (w5232:string)
                    n2874 = Concatenate Strings(w5219, w5243, w5219, w5242, w5219, w5241) -> (w5231:string)
                    n2875 = Concatenate Strings(w5219, w5286, w5219, w5285, w5219, w5284) -> (w5240:string)
                    n2876 = Concatenate Strings(w5219, w5266, w5219, w5265, w5219, w5264) -> (w5236:string)
                    n2877 = Concatenate Strings(w5219, w5281, w5219, w5280, w5219, w5279) -> (w5239:string)
                    n2878 = Concatenate Strings(w5219, w5278, w5219, w5277, w5219, w5274) -> (w5238:string)
                    n2879 = Concatenate Strings(w5219, w5271, w5219, w5270, w5219, w5269) -> (w5237:string)
